vi "FPGA myRIO Ultrasound.vi"() -> ()   [LabVIEW 2013]
uses:
  <vilib>/eio/EIONode/EIONode.xnode
  <vilib>/rvi/eio/common/nirviEmuTemplateMethod_errors.vi
panel:
  in  "Trigger pulse interval (mSec)":u32=200
  out "Time of flight (uS)":u32
  in  "stop":bool
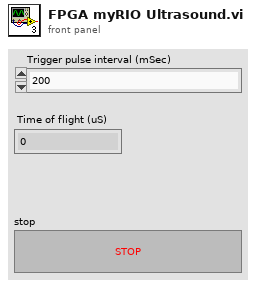
[diagram p1: front panel]
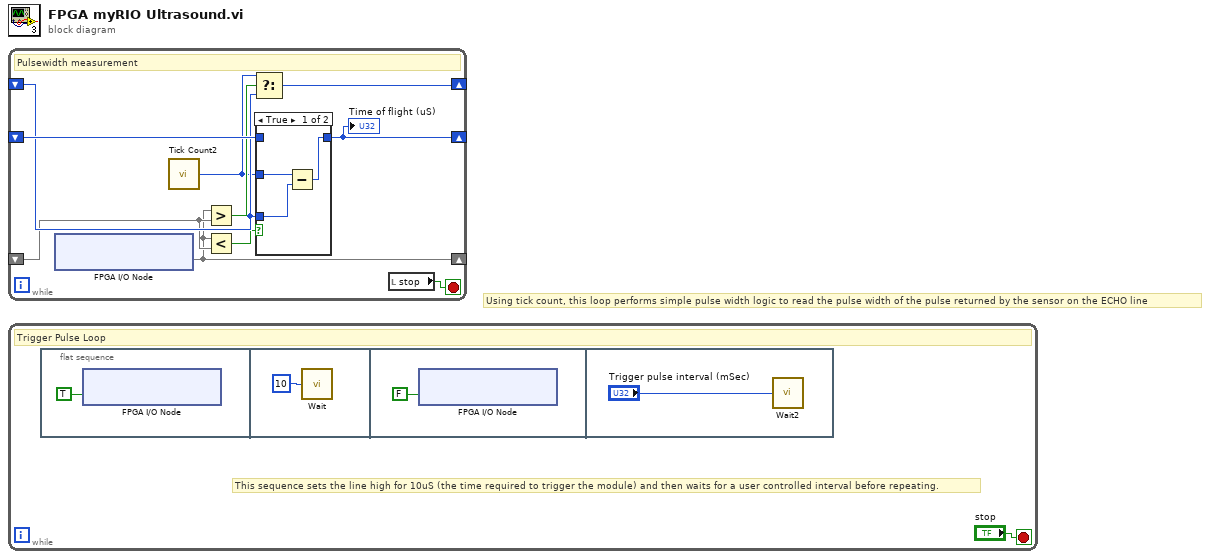
[diagram p0: block diagram]
diagram:
  # "Using tick count, this loop performs simple pulse width logic to read the pulse width of the pulse returned by the sensor on the ECHO line"
  n1 = while "Pulsewidth Measurement + Sound Output" {
    shift-left: _ -> [w10]
    shift-right: [w4] -> _
    shift-left: _ -> [w9]
    shift-right: [w8] -> _
    shift-left: _ -> [w6]
    shift-right: [w3] -> _
    stop <- w1 stop-if-true
    # "Pulsewidth measurement"
    n2 = xnode "FPGA I/O Node"() -> ("ConnectorC/DIO3"=w3)  [unwired: 1 in, 1 out]
    n3 = call "Tick Count2"() -> ("Tick Count(uSec)"=w2:u32)
    n4 = Greater?(x=w3, y=w6) -> (0:w7:bool)
    n5 = Less?(x=w3, y=w6) -> (x < y?=w5:bool)
    n6 = Select(t=w2, s=w7, f=w9) -> (s? t:f=w8:u32)
    n7 = case shown="True" w5 {
      tunnel: w10 -> [_ w14]
      tunnel: w2 -> [w11 _]
      tunnel: w9 -> [w12 _]
      tunnel: [w13 w14] -> w4
      frame True {
        n8 = Subtract(x=w11, y=w12) -> (x-y=w13:u32)
      }
      frame False {
      }
    }
    "Time of flight (uS)" <- w4
    n9 = local read "stop"() -> (w1:bool)
  }
  n10 = while {
    stop <- "stop" stop-if-true
    # "This sequence sets the line high for 10uS (the time required to trigger the module) and then waits for a user controlled interval before repeating."
    # "Trigger Pulse Loop"
    n11 = flat-sequence {
      frame #0 {
        n12 = xnode "FPGA I/O Node"("ConnectorC/DIO7"=TRUE ("ConnectorC/DIO6")) -> ()  [unwired: 1 in, 1 out]
      }
      frame #1 {
        n13 = call "Wait"("Count(uSec)"=u32 10) -> ()  [unwired: 1 out]
      }
      frame #2 {
        n14 = xnode "FPGA I/O Node"("ConnectorC/DIO7"=FALSE ("ConnectorC/DIO6")) -> ()  [unwired: 1 in, 1 out]
      }
      frame #3 {
        n15 = call "Wait2"("Count(mSec)"="Trigger pulse interval (mSec)") -> ()  [unwired: 1 out]
      }
    }
  }
